vi "Instantiate Look Up Table.vi"(8 "error in (no error)":errorcluster) -> (0 "error out":errorcluster, 3 "Look Up Table out":refnum<class "Look Up Table.lvclass">)   [LabVIEW 2016, in "Stream Look Up Table.lvlib" / "Look Up Table.lvclass"]
doc: "--\nCopyright © 2017 Composed SystemsI All rights reserved.\n\nAuthor: Jon McBee <jon.mcbee@composed.io>\n\nThis library is provided \"AS IS\" ,WITHOUT WARRANTIES OR\nCONDITIONS OF ANY KIND, either express or implied.\n\nComposed Systems -- composed.io\n\nStream 0.0.1.1\nJon McBee - Composed Systems\nCopyright (c) 2017, Composed Systems"
uses:
  <userlib>/Composed Systems/Stream/Look Up Table/Look Up Table/Look Up Table.lvclass
  <userlib>/Composed Systems/Stream/Look Up Table/Look Up Table/Look Up Table.lvclass/Look Up Table.ctl
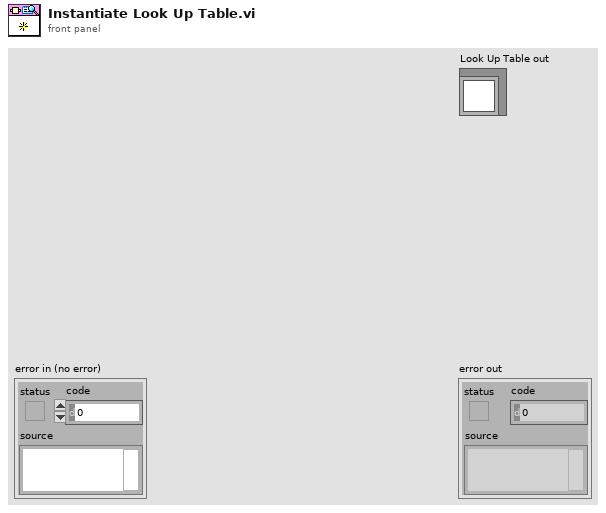
[diagram p1: front panel]
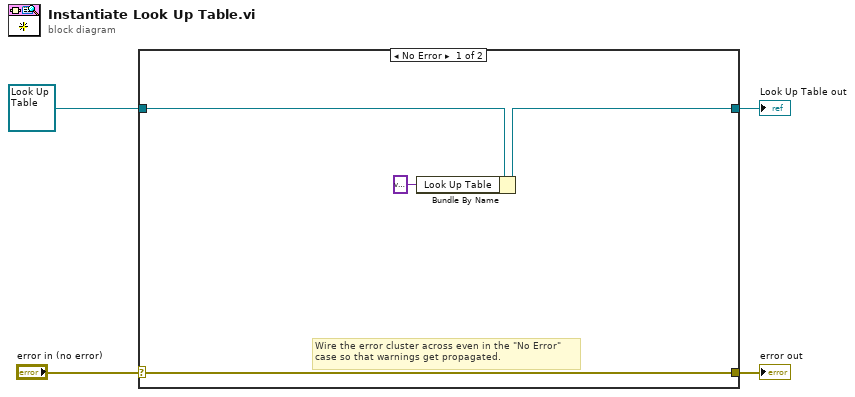
[diagram p0: block diagram]
diagram:
  n1 = case shown="No Error" "error in (no error)" {
    selector: "error in (no error)" -> [w8 w10]
    tunnel: [w8 w10] -> w3
    tunnel: [w6 w9] -> w1
    tunnel: refnum<class "Look Up Table.lvclass"> refnum ("Look Up Table in") -> [w7 w9]
    frame No Error {
      # "Wire the error cluster across even in the \"No Error\"\ncase so that warnings get propagated."
      n2 = Bundle By Name(cluster=w7, "Look Up Table"=variant) -> (w6:refnum<class "Look Up Table.lvclass">)
    }
    frame Error {
    }
  }
  "error out" <- w3
  "Look Up Table out" <- w1
